vi "Read sequence state.vi"(8 "error in (no error)":errorcluster, 11 "Change Sequence State MSG in":refnum<class "Change Sequence State MSG.lvclass">) -> (0 "error out":errorcluster, 2 "sequence state":T1, 3 "Change Sequence State MSG out":refnum<class "Change Sequence State MSG.lvclass">)   [LabVIEW 2017, in "Controller.lvlib" / "Change Sequence State MSG.lvclass"]
uses:
  Change Sequence State MSG.lvclass
  Sequencer/sequenceState.ctl
  Change Sequence State MSG.lvclass/Change Sequence State MSG.ctl
  Controller.lvlib
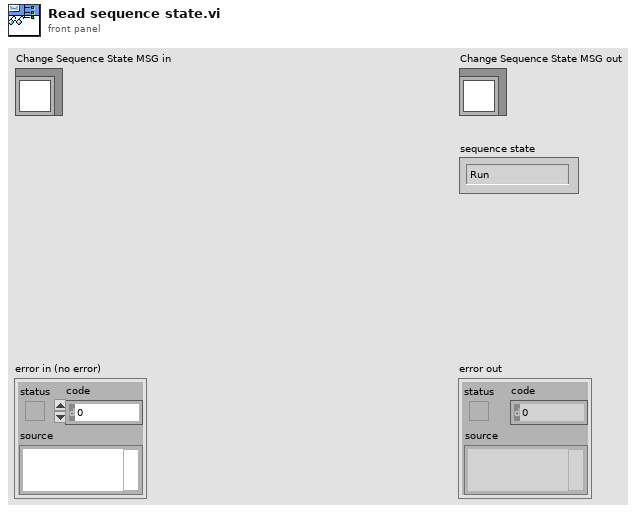
[diagram p1: front panel]
types:
  T1 = typedef "Controller.lvlib/sequenceState.ctl" = enum16{"Run", "Pause", "Reset", "Reload", "Stop"}
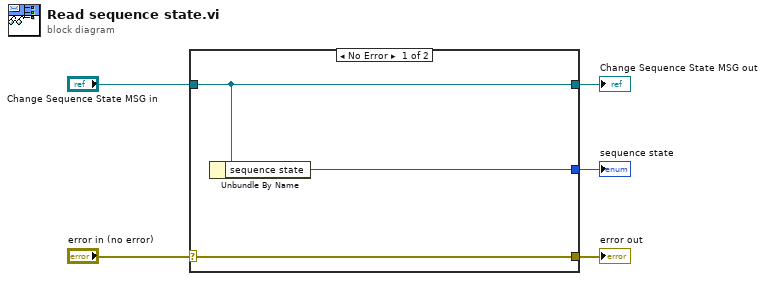
[diagram p0: block diagram]
diagram:
  n1 = case shown="No Error" "error in (no error)" {
    selector: "error in (no error)" -> [w8 w9]
    tunnel: [w8 w9] -> w4
    tunnel: [w7 w10] -> w2
    tunnel: "Change Sequence State MSG in" -> [w7 w10]
    tunnel: [w6 _] -> w1
    frame No Error {
      n2 = Unbundle By Name(w7) -> ("sequence state"=w6:T1)
    }
    frame Error {
    }
  }
  "error out" <- w4
  "Change Sequence State MSG out" <- w2
  "sequence state" <- w1
